vi "test Sec-WebSocket-Key logic.vi"() -> ()   [LabVIEW 2017]
panel:
  out "SHA-1":string
  out "Sec-WebSocket-Accept":string
  in  "Sec-WebSocket-Key":string
  # "https://developer.mozilla.org/en-US/docs/Web/API/WebSockets_API/Writing_WebSocket_servers\nKey: dGhlIHNhbXBsZSBub25jZQ==\nAccept: s3pPLMBiTxaQ9kYGzzhZRbK+xOo="
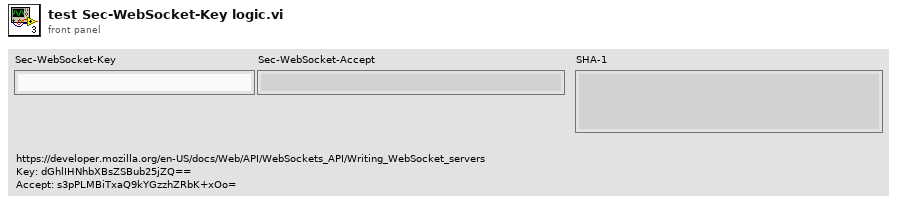
[diagram p1: front panel]
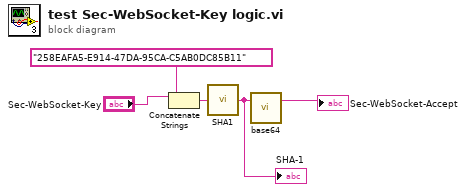
[diagram p0: block diagram]
diagram:
  n1 = Concatenate Strings("Sec-WebSocket-Key", "258EAFA5-E914-47DA-95CA-C5AB0DC85B11" ("trimmed string")) -> (w5:string)
  n2 = call "SHA1.vi"("String"=w5) -> ("SHA1"=w1:string)
  "SHA-1" <- w1
  n3 = call "base64.vi"("string in"=w1) -> ("base64 out"=→"Sec-WebSocket-Accept":string)  [unwired: 1 in, 1 out]
